vi "ConvertStepsmm.vi"(6 "Conversion: T: pas->mm\n                      F: mm->pas":bool, 9 "Input en pas":i32[](array[numeric]), 10 "Input en mm":dbl[](array[numeric]), 11 "Facteur de conversion\n en µm/pas":dbl[](array[numeric])) -> (1 "Output en mm":dbl[](array[numeric]) format="%#_6f", 2 "output en pas":i32[](array[numeric]))   [LabVIEW 2012]
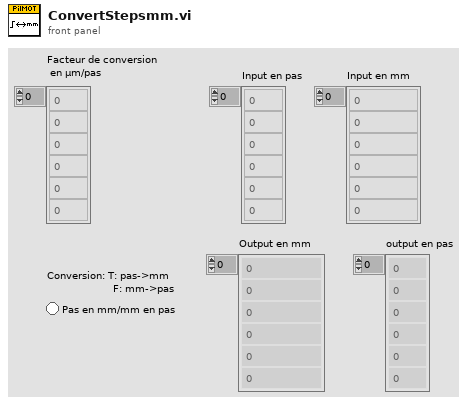
[diagram p1: front panel]
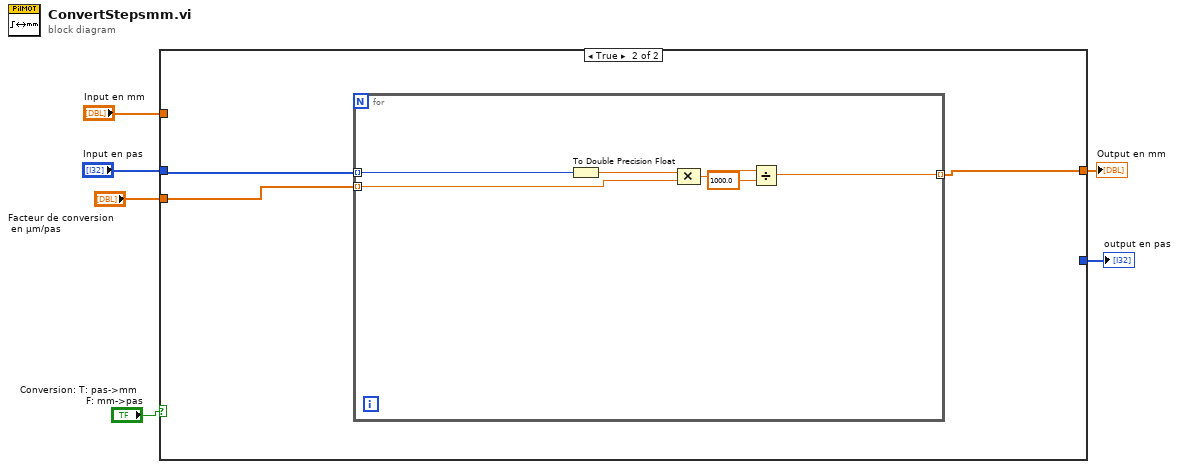
[diagram p0: block diagram]
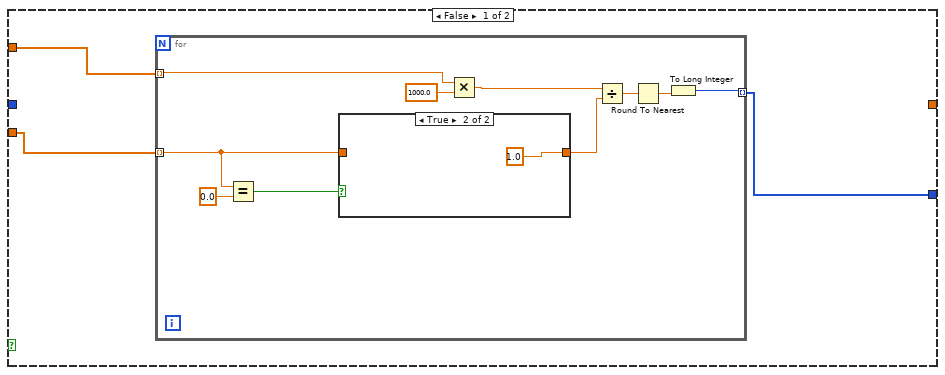
[diagram p2: hidden frame]
diagram:
  n1 = case shown="True" "Conversion: T: pas->mm\n                      F: mm->pas" {
    tunnel: "Input en pas" -> [_ w24]
    tunnel: "Facteur de conversion\n en µm/pas" -> [w8 w23]
    tunnel: "Input en mm" -> [w9 _]
    tunnel: [w7 _] -> w2
    tunnel: [_ w22] -> w1
    frame False {
      n2 = for {
        tunnel: [w12] -> w7 mode=indexing
        tunnel: w9 -> [w11] mode=indexing
        tunnel: w8 -> [w10] mode=indexing
        n3 = Equal?(x=w10, y=0.0) -> (x = y?=w16:bool)
        n4 = case shown="True" w16 {
          tunnel: [w20 1.0 ("facteur de conversion en µm/pas")] -> w15
          tunnel: w10 -> [w20 _]
          frame False {
          }
          frame True {
          }
        }
        n5 = Multiply(x=w11, y=1000.0) -> (x*y=w13:dbl)
        n6 = Divide(x=w13, y=w15) -> (x/y=w19:dbl)
        n7 = Round To Nearest(number=w19) -> (nearest integer value=w18:dbl)
        n8 = To Long Integer(number=w18) -> (32bit integer=w12:i32)
      }
    }
    frame True {
      n9 = for {
        tunnel: [w27] -> w22 mode=indexing
        tunnel: w24 -> [w29] mode=indexing
        tunnel: w23 -> [w28] mode=indexing
        n10 = To Double Precision Float(number=w29) -> (double precision float=w30:dbl)
        n11 = Compound Arithmetic op=MULTIPLY(w30, w28) -> (w26:dbl)
        n12 = Divide(x=w26, y=1000.0) -> (x/y=w27:dbl)
      }
    }
  }
  "output en pas" <- w2
  "Output en mm" <- w1
